vi "Get Internal Xp.vi"(8 "error in":errorcluster, 11 "VISA resource name in":refnum<visa-resource-name>) -> (0 "error out":errorcluster, 1 "InternalXp (out)":dbl, 3 "VISA resource name out":refnum<visa-resource-name>)   [LabVIEW 2018, in "JULABO DeviceDriver.lvlib"]
doc: "This VI returns the Proportional component <B>Xp</B> in case of internal temperature control."
uses:
  JULABO DeviceDriver.lvlib
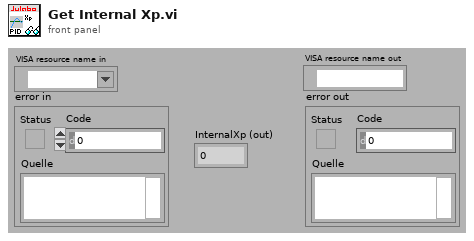
[diagram p1: front panel]
types:
  T1 = typedef "JULABO DeviceDriver.lvlib/InstrumentType.ctl" = enum8{"Default", "FC-Series", "HT30/HT60", "LC4"}
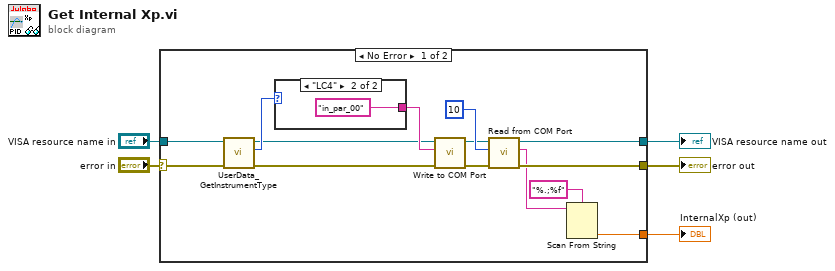
[diagram p0: block diagram]
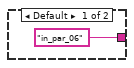
[diagram p2: hidden frame]
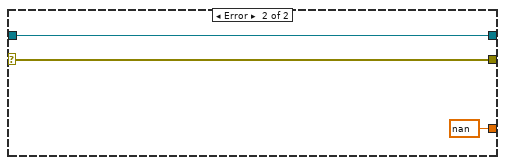
[diagram p3: hidden frame]
diagram:
  n1 = case shown="No Error" "error in" {
    selector: "error in" -> [w8 w23]
    tunnel: "VISA resource name in" -> [w9 w24]
    tunnel: [w19 w23] -> w4
    tunnel: [w18 w24] -> w3
    tunnel: [w14 nan] -> w1
    frame No Error {
      n2 = call "UserData_GetInstrumentType.vi"("Fehler (Eingang)"=w8, "VISA resource name in"=w9) -> ("Fehler (Ausgang)"=w11:errorcluster, "InstrumentType"=w12:T1, "VISA resource name out"=w10:refnum<visa-resource-name>)  [unwired: 3 in]
      n3 = case shown="\"LC4\"" w12 {
        tunnel: ["in_par_06" "in_par_00"] -> w13
        frame Default {
        }
        frame "LC4" {
        }
      }
      n4 = call "Write to COM Port.vi"("error in"=w11, "Command (input)"=w13, "VISA resource name in"=w10) -> ("error out"=w6:errorcluster, "VISA resource name out"=w7:refnum<visa-resource-name>)  [unwired: 7 in]
      n5 = call "Read from COM Port.vi"("error in"=w6, "Byte to Read (-1:All)"=10 ("Anzahl der Byte"), "VISA resource name in"=w7) -> ("error out"=w19:errorcluster, "String (output)"=w16:string, "VISA resource name out"=w18:refnum<visa-resource-name>)  [unwired: 5 in, 1 out]
      n6 = Scan From String(format string="%.;%f" ("Format-String"), input string=w16) -> (output 1=w14:dbl)  [unwired: 3 in, 3 out]
    }
    frame Error {
    }
  }
  "VISA resource name out" <- w3
  "error out" <- w4
  "InternalXp (out)" <- w1
